vi "Waage final version.vi"() -> ()   [LabVIEW 2020]
uses:
  <vilib>/Utility/error.llb/DialogType.ctl
panel:
  out "Fehlermeldungen":string=" ANWEISUNGEN:\r\rAllgemeine Nutzung:  Bei der Benutzung von SubVIs, die mit den Anschlüssen \"Fehler(Eingang)\" und \"Fehler(Ausgang)\" arbeiten, platzieren Sie diesen Handler dort, wo Sie den Benutzer auf aufgetretene Fehler hinweisen möchten. In der Regel wird er am Ende eines Datenpfads als letzte Aktion des Programms aufgerufen.  Wenn der Fehlerstatus einen Fehler angibt, erzeugt der Handler eine Nachricht, die den Fehler und dessen Ursprung beschreibt.  Ist Dialogtyp = 1 (Standardeinstellung), wird die Fehlermeldung angezeigt und der Benutzer kann diese bestätigen.  Ist Dialogtyp = 2, kann der Benutzer die Meldung bestätigen oder die Programmausführung abbrechen. Der Abbruch eines Programms mit aktiver I/O wird jedoch nicht empfohlen.  Ist der Dialogtyp = 0, wird keine Meldung angezeigt; dieser Modus wird verwendet, um Fehler programmatisch zu behandeln. Aus diesem Grunde sind auch die Fehlerausgangs-Cluster mit individuellen Anschlüssen verbunden.  \r\rAndere Nutzungsmöglichkeit:\n\r\nLokales Testen.  Um einen Fehlercode eines SubVIs oder einer Funktion zu testen, die nicht mit den Fehleranschlüssen arbeitet, können der Fehlercode und ein String für \"Quelle\" mit den lokalen Eingängen \"Fehlercode\" und \"Quelle\" verbunden werden.  Wenn der Fehlerstatus keinen Fehler anzeigt und der Fehlercode ungleich 0 ist, werden der lokale Code und String \"Quelle\" ersetzt und \"Fehler?\" lautet TRUE (FEHLER)." caption="Nachricht"
  out "Gelöschte Elemente \ndes Angehängten \nVektors":dbl[][](array[numeric])
  out "Angehängter Vektor":dbl[][](array[numeric])
  out "Größe(n) \ndes Ange-\nhängten \nVektors":i32
  out "Vektor des neuen \nWertepaares":dbl[](array[numeric])
  out "Dauer der Messung [s]":dbl
  in  "Kalibrierung [2000 g]":bool
  in  "Tara":bool
  out "Start der Messung":timestamp
  out "Waage":cluster{"Y":dbl[], "Y":dbl[]}[](graph)
  in  "Reset Waage":bool caption="Reset"
  out "Aktueller Wert [g]":dbl
  in  "Waage":refnum<visa-resource-name>="COM11"
  # "Debug Area"
  # "Konfiguration"
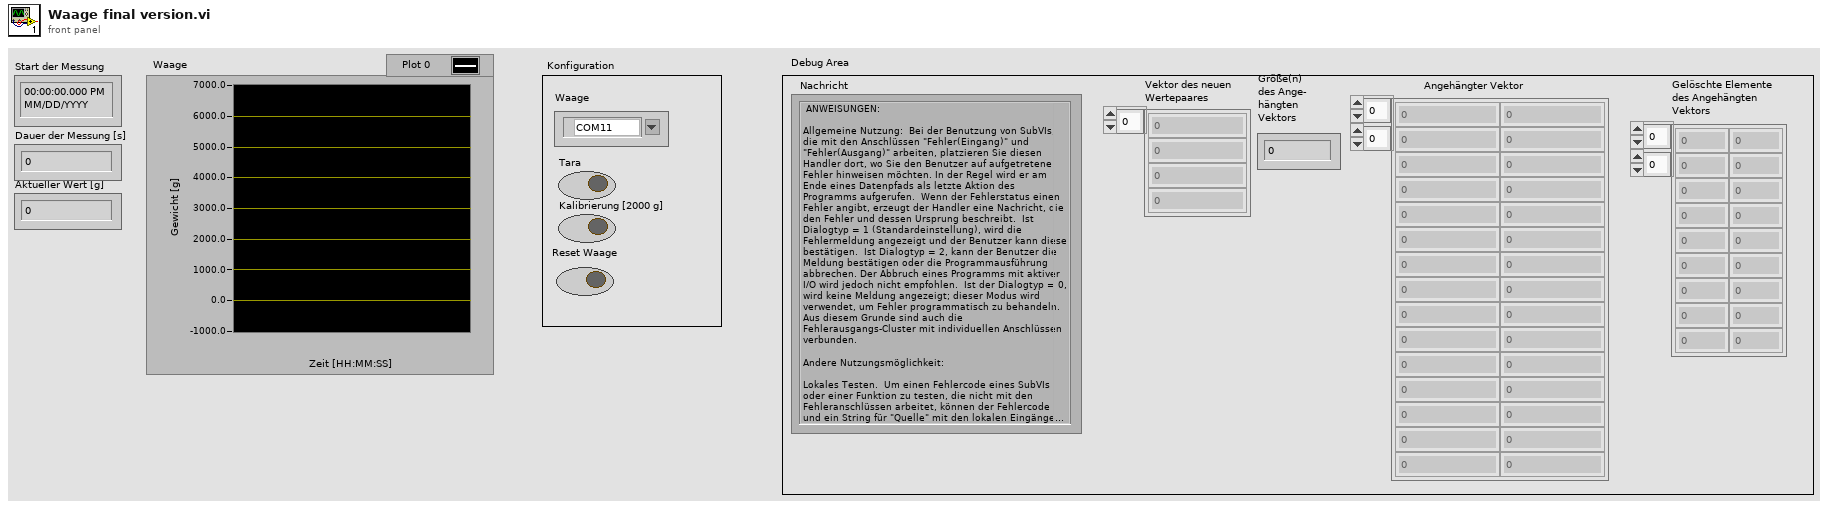
[diagram p1: front panel]
types:
  T1 = typedef "DialogType.ctl" = u16
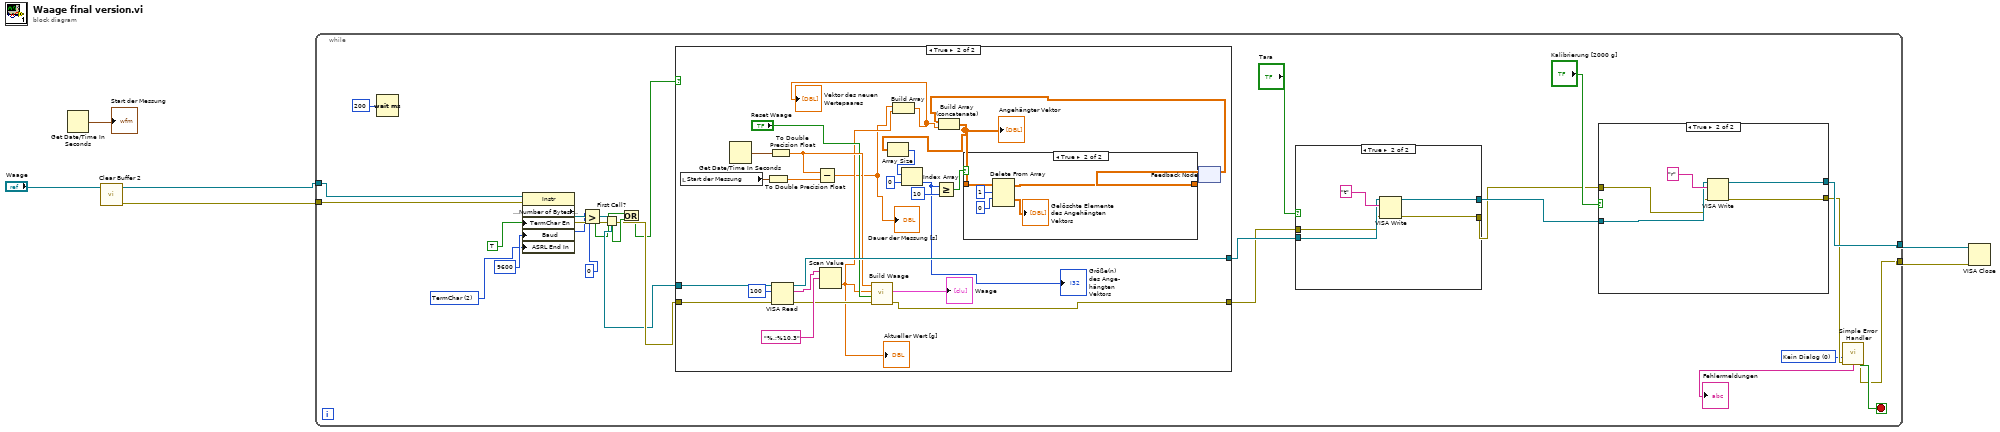
[diagram p0: block diagram]
diagram:
  n1 = Get Date/Time In Seconds() -> (seconds since 1Jan1904=→"Start der Messung":timestamp)
  n2 = call "Clear Buffer 2.vi"("VISA-Referenz (Eingang)"="Waage") -> ("Fehler (Ausgang)"=w3:errorcluster, "VISA-Referenz (Ausgang)"=w4:refnum<visa-resource-name>)  [unwired: 9 in]
  n3 = while {
    tunnel: w4 -> [w24]
    tunnel: w3 -> [w23]
    tunnel: [w13] -> w2
    tunnel: [w11] -> w1
    stop <- w26 stop-if-true
    w8 = T1 0 items=["Kein Dialog", "OK-Meldung", "Dialog zum Fortsetzen oder Anhalten", "OK-Meldung + Warnungen", "Weiter/Stopp + Warnung"] ("type of dialog (OK msg:1)")
    w9 = u16 2 items=["None", "Last Bit", "TermChar"] ("Serial Settings:End Mode for Reads")
    n4 = Wait (ms)(milliseconds to wait=u32 200) -> ()  [unwired: 1 out]
    n5 = property class="Instr"(reference=w24, error in=w23, "TermChar En"=TRUE, "Baud"=u32 9600 ("Serial Settings:Baud Rate"), "ASRL End In"=w9) -> (reference out=w28:refnum<visa-resource-name>, error out=w29:errorcluster, "Serial Settings:Number of Bytes at Serial Port"=w22:u32)
    n6 = Greater?(x=w22, y=u32 0) -> (0:w20:bool)
    n7 = First Call?() -> (First Call?: T/F=w30:bool)
    n8 = Or(x=w20, y=w30) -> (x .or. y?=w27:bool)
    n9 = case shown="True" w27 {
      tunnel: w28 -> [w47 w72]
      tunnel: w29 -> [w46 w71]
      tunnel: [w47 w70] -> w18
      tunnel: [w46 w65] -> w17
      frame False {
      }
      frame True {
        n10 = local read "Start der Messung"() -> (w64:timestamp)
        n11 = Get Date/Time In Seconds() -> (seconds since 1Jan1904=w68:timestamp)
        n12 = To Double Precision Float(number=w64) -> (double precision float=w63:dbl)
        n13 = To Double Precision Float(number=w68) -> (double precision float=w62:dbl)
        n14 = VISA Read(VISA resource name=w72, byte count=u32 100 ("Byte-Anzahl"), error in (no error)=w71) -> (VISA resource name out=w70:refnum<visa-resource-name>, read buffer=w59:string, error out=w66:errorcluster)  [unwired: 1 out]
        n15 = Subtract(x=w62, y=w63) -> (x-y=w56:dbl)
        "Dauer der Messung [s]" <- w56
        n16 = Scan Value(string=w59, format string="%.;%10.3") -> (value=w57:dbl)  [unwired: 1 in, 1 out]
        "Aktueller Wert [g]" <- w57
        n17 = call "Build Waage"("error in (no error)"=w66, "Reset"="Reset Waage", "Y Input"=w57, "X Input"=w62) -> ("error out"=w65:errorcluster, "XY Graph"=→"Waage":cluster{"X":dbl[], "Y":dbl[]}[])  [unwired: 6 in]
        n18 = Build Array(w56, w57) -> (w55:dbl[])
        "Vektor des neuen \nWertepaares" <- w55
        n19 = feedback #1() -> (w54:dbl[][])  [unwired: 1 in]
        n20 = Build Array (concatenate)(w54, w55) -> (w53:dbl[][])
        "Angehängter Vektor" <- w53
        n21 = Array Size(array=w53) -> (size(s)=w52:i32[])
        n22 = Index Array(array=w52, index=0 ("Index")) -> (element=w48:i32)
        "Größe(n) \ndes Ange-\nhängten \nVektors" <- w48
        n23 = Greater Or Equal?(x=w48, y=10) -> (x >= y?=w50:bool)
        n24 = case shown="True" w50 {
          tunnel: w53 -> [w73 w78]
          tunnel: [w73 w77] -> w58
          frame False {
          }
          frame True {
            n25 = Delete From Array(array=w78, length=1 ("Länge"), index (row)=0 ("Index")) -> (deleted portion=→"Gelöschte Elemente \ndes Angehängten \nVektors":dbl[][], array with subset deleted=w77:dbl[][])  [unwired: 1 in]
          }
        }
        n26 = feedback-in #1(w58) -> ()
      }
    }
    n27 = case shown="True" "Tara" {
      tunnel: w18 -> [w39 w44]
      tunnel: w17 -> [w40 w43]
      tunnel: [w39 w42] -> w15
      tunnel: [w40 w41] -> w14
      frame False {
      }
      frame True {
        n28 = VISA Write(VISA resource name=w44, write buffer="t" ("Schreibpuffer"), error in (no error)=w43) -> (VISA resource name out=w42:refnum<visa-resource-name>, error out=w41:errorcluster)  [unwired: 1 out]
      }
    }
    n29 = case shown="True" "Kalibrierung [2000 g]" {
      tunnel: w15 -> [w32 w37]
      tunnel: w14 -> [w33 w36]
      tunnel: [w32 w35] -> w13
      tunnel: [w33 w34] -> w12
      frame False {
      }
      frame True {
        n30 = VISA Write(VISA resource name=w37, write buffer="r" ("Schreibpuffer"), error in (no error)=w36) -> (VISA resource name out=w35:refnum<visa-resource-name>, error out=w34:errorcluster)  [unwired: 1 out]
      }
    }
    n31 = call <vilib>:"Simple Error Handler.vi"("type of dialog (OK msg:1)"=w8, "error in (no error)"=w12) -> ("error?"=w26:bool, "error out"=w11:errorcluster, "message"=→"Fehlermeldungen":string)  [unwired: 5 out]
  }
  n32 = VISA Close(VISA resource name=w2, error in (no error)=w1) -> ()  [unwired: 1 out]
